vi "Get SLSC Switch CD Description.vi"(8 "error in (no error)":errorcluster, 11 "SLSC Sw Custom Device Ref in":T1 format="%.0x") -> (0 "error out":errorcluster, 2 "Description":string, 3 "SLSC Sw Custom Device Ref out":T1 format="%.0x")   [LabVIEW 2017, in "SLSC Switch Scripting.lvlib"]
uses:
  SLSC Switch Scripting.lvlib
  <vilib>/NI Veristand/Custom Device API/Custom Device Item Ref.ctl
  <vilib>/NI VeriStand/Custom Device API/Custom Device API.lvlib
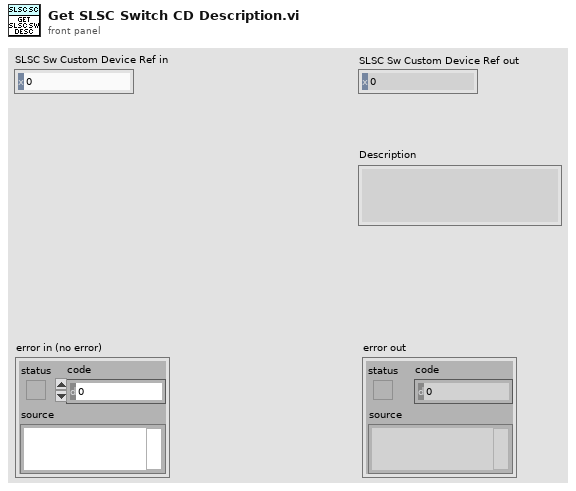
[diagram p1: front panel]
types:
  T1 = typedef "Custom Device API.lvlib/Custom Device Item Ref.ctl" = u64
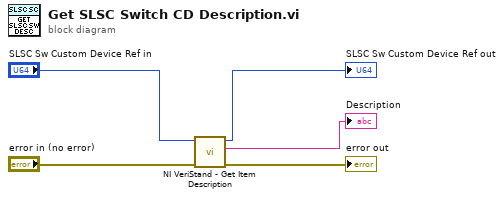
[diagram p0: block diagram]
diagram:
  n1 = call <vilib>:"NI VeriStand - Get Item Description.vi"("error in (no error)"="error in (no error)", "Item Ref in"="SLSC Sw Custom Device Ref in") -> ("error out"=→"error out":errorcluster, "Description"=→"Description":string, "Item Ref out"=→"SLSC Sw Custom Device Ref out":T1)  [unwired: 6 in, 1 out]
